vi "Entry.vi"(8 "error in (no error)":errorcluster, 11 "New State":refnum<class "Started.lvclass">) -> (0 "error out":errorcluster, 3 "State out":refnum<class "Started.lvclass">)   [LabVIEW 2013, in "Command State Actor.lvlib" / "Started.lvclass"]
doc: "This is an abstract method. Override this method to define the behavior when you enter the state."
uses:
  Started.lvclass
  Command State Actor.lvclass
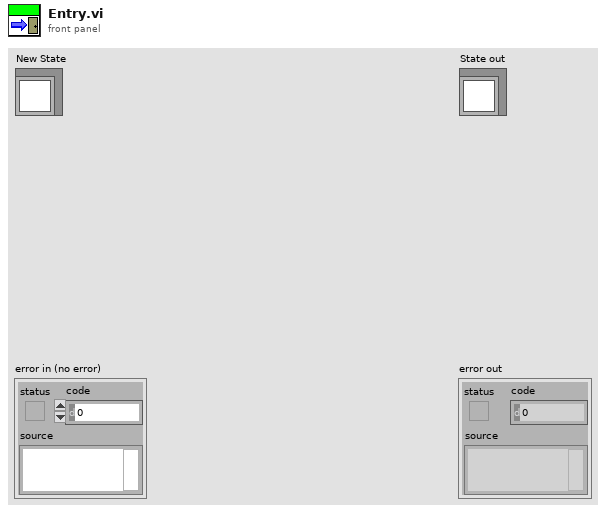
[diagram p1: front panel]
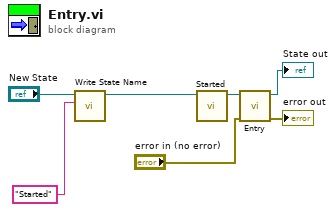
[diagram p0: block diagram]
diagram:
  n1 = call-dynamic "Write State Name.vi"("State Name"="Started", "Command State Actor in"="New State") -> ("Command State Actor out"=w3:refnum<class "Started.lvclass">)  [unwired: 8 in, 1 out]
  n2 = call-dynamic "Started.vi"("Command State Actor in"=w3) -> ("Command State Actor out"=w2:refnum<class "Started.lvclass">)  [unwired: 9 in, 1 out]
  n3 = call-parent "Entry.vi"("error in (no error)"="error in (no error)", "New State"=w2) -> ("error out"=→"error out":errorcluster, "State out"=→"State out":refnum<class "Started.lvclass">)  [unwired: 8 in]
